vi "I2C Write.vi"(9 "data":u8, 10 "intAddress":u8, 11 "deviceID":u8) -> (3 "function return":u32)   [LabVIEW 2018, in "Copy of Andor SDK.lvlib"]
doc: "EXPNETTYPE unsigned int WINAPI I2CWrite(BYTE deviceID, BYTE intAddress, BYTE data);"
uses:
  Copy of Andor SDK.lvlib
  <userlib>/Andor SDK/ATMCD32D.dll
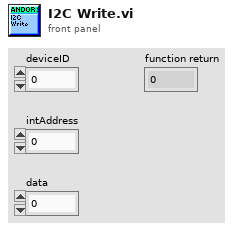
[diagram p1: front panel]
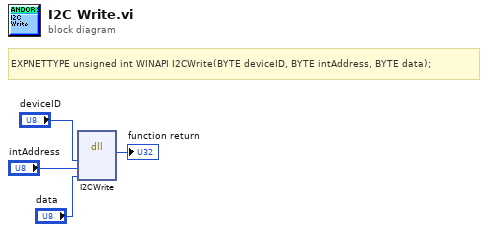
[diagram p0: block diagram]
diagram:
  # "EXPNETTYPE unsigned int WINAPI I2CWrite(BYTE deviceID, BYTE intAddress, BYTE data);"
  n1 = dll-call lib="C:/Program Files (x86)/National Instruments/LabVIEW 2018/user.lib/Andor SDK/ATMCD32D.*" fn="I2CWrite"("deviceID"="deviceID", "intAddress"="intAddress", "data"="data") -> (→"function return":u32)  [unwired: 6 in, 2 out]
